vi "DSF.Shared.Configuration.Plugin.Create.vi"(8 "error in (no error)":errorcluster, 10 "Plugin Configuration cluster":T1={"name"="", "class"="", "cycle timing"={"priority"=0, "decimation"=1, "offset"=0}, "Transfer Groups"=[], "settings"=[]}, 11 "Plugin Configuration in":refnum<class "DSF.Shared.Configuration.Plugin.lvclass">) -> (0 "error out":errorcluster, 3 "Plugin Configuration out":refnum<class "DSF.Shared.Configuration.Plugin.lvclass">)   [LabVIEW 2017, in "DSF.Engine.lvlib" / "DSF.Shared.Configuration.Plugin.lvclass"]
uses:
  DSF.Shared.Configuration.Plugin.lvclass
  DSF Configuration API/1.0.0/Public/Controls/DSF Engine Plugin Configuration.ctl
  DSF Configuration API/1.0.0/Public/Controls/DSF Timing Info.ctl
  DSF Configuration API/1.0.0/Public/Controls/DSF Engine Transfer Group Configuration.ctl
  DSF Configuration API/1.0.0/Public/Controls/DSF Direction.ctl
  DSF Configuration API/1.0.0/Public/Controls/DSF Engine Transfer Configuration.ctl
  DSF Configuration API/1.0.0/Public/Controls/DSF Byte Order.ctl
  DSF Configuration API/1.0.0/Public/Controls/DSF Engine Channel Configuration.ctl
  DSF Configuration API/1.0.0/Public/Controls/DSF Data Type.ctl
  DSF Configuration API/1.0.0/Public/Controls/DSF Settings Info.ctl
  Transfer Group/DSF.Shared.Configuration.Transfer Group.lvclass
  DSF.Shared.Configuration.Plugin.lvclass/DSF.Shared.Configuration.Plugin.ctl
  DSF Configuration API/1.0.0/DSF Configuration API.lvlib
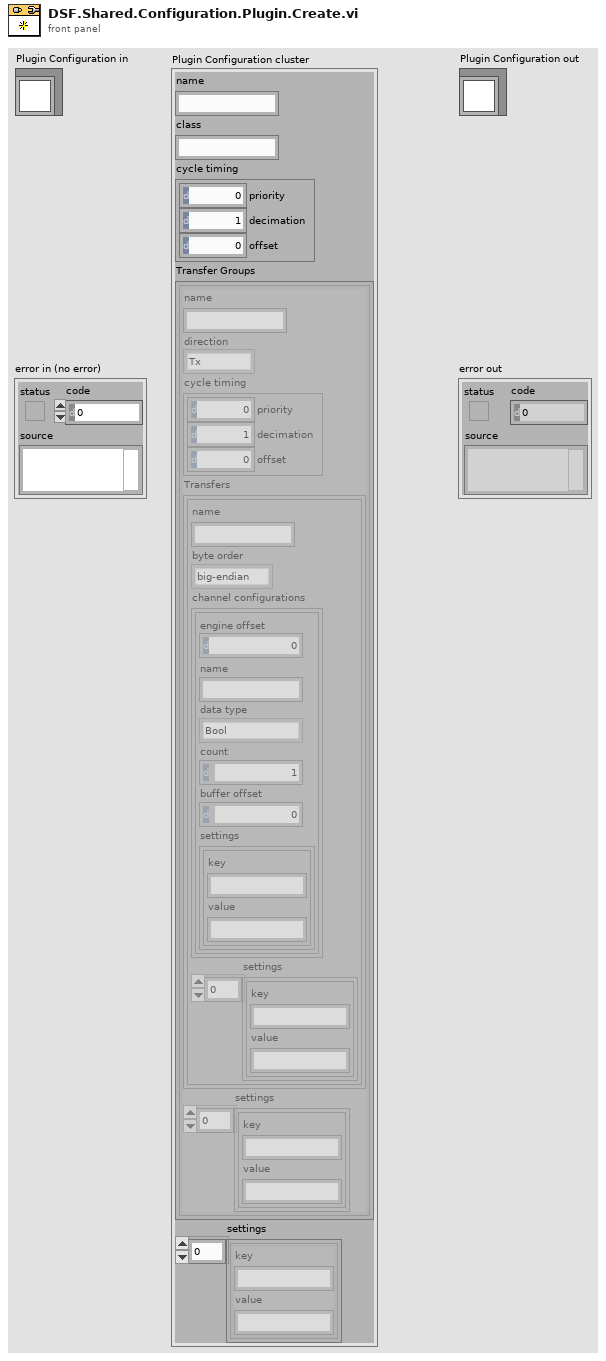
[diagram p1: front panel]
types:
  T1 = typedef "DSF Configuration API.lvlib/DSF Engine Plugin Configuration.ctl" = cluster{"name":string, "class":string, "cycle timing":T2, "Transfer Groups":T3[], "settings":T9}
  T2 = typedef "DSF Configuration API.lvlib/DSF Timing Info.ctl" = cluster{"priority":u64, "decimation":u64, "offset":u64}
  T3 = typedef "DSF Configuration API.lvlib/DSF Engine Transfer Group Configuration.ctl" = cluster{"name":string, "direction":T4, "cycle timing":T2, "Transfers":T5[], "settings":T9}
  T4 = typedef "DSF Configuration API.lvlib/DSF Direction.ctl" = enum8{"Tx", "Rx"}
  T5 = typedef "DSF Configuration API.lvlib/DSF Engine Transfer Configuration.ctl" = cluster{"name":string, "byte order":T6, "channel configurations":T7[], "settings":T9}
  T6 = typedef "DSF Configuration API.lvlib/DSF Byte Order.ctl" = enum8{"big-endian", "little-endian"}
  T7 = typedef "DSF Configuration API.lvlib/DSF Engine Channel Configuration.ctl" = cluster{"engine offset":u64, "name":string, "data type":T8, "count":u64, "buffer offset":u64, "settings":T9}
  T8 = typedef "DSF Configuration API.lvlib/DSF Data Type.ctl" = enum8{"Bool", "SGL", "DBL", "I8", "I16", "I32", "I64", "U8", "U16", "U32", "U64"}
  T9 = typedef "DSF Configuration API.lvlib/DSF Settings Info.ctl" = cluster{"key":string, "value":string}[]
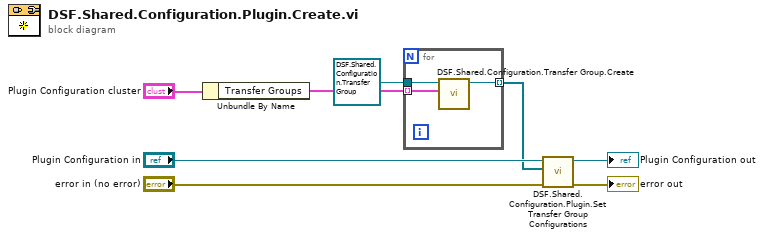
[diagram p0: block diagram]
diagram:
  n1 = Unbundle By Name("Plugin Configuration cluster") -> ("Transfer Groups"=w3:T3[])
  n2 = for {
    tunnel: w3 -> [w10] mode=indexing
    tunnel: refnum<class "DSF.Shared.Configuration.Transfer Group.lvclass"> refnum ("DSF.Shared.lvlib:Transfer Group Configuration") -> [w9]
    tunnel: [w8] -> w1 mode=indexing
    n3 = call "DSF.Shared.Configuration.Transfer Group.Create.vi"("Transfer Group Configuration"=w10, "Transfer Group Configuration in"=w9) -> ("Transfer Group Configuration out"=w8:refnum<class "DSF.Shared.Configuration.Transfer Group.lvclass">)  [unwired: 8 in, 1 out]
  }
  n4 = call "DSF.Shared.Configuration.Plugin.Set Transfer Group Configurations.vi"("Transfer Group Configurations"=w1, "Plugin Configuration in"="Plugin Configuration in") -> ("Plugin Configuration out"=→"Plugin Configuration out":refnum<class "DSF.Shared.Configuration.Plugin.lvclass">)  [unwired: 9 in]
  "error out" <- "error in (no error)"
